vi "网络_构建url.vi"(10 "url":string, 11 "参数":string[](array[string])) -> (3 "结果url":string)   [LabVIEW 2014]
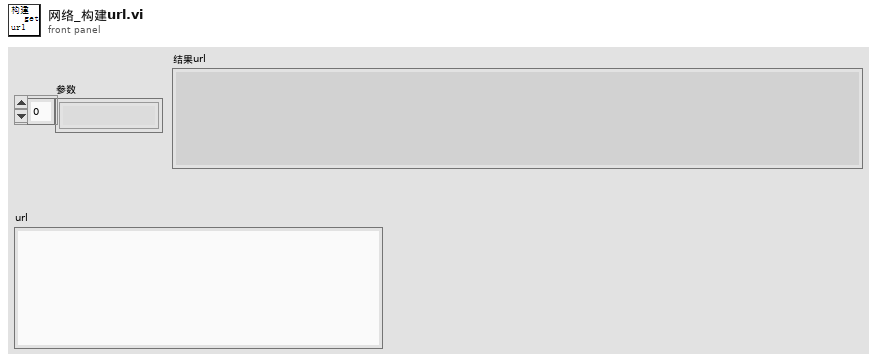
[diagram p1: front panel]
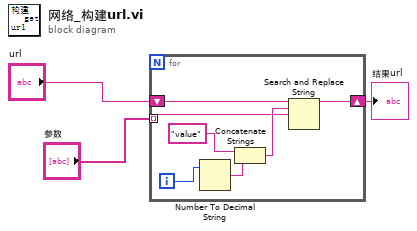
[diagram p0: block diagram]
diagram:
  n1 = for {
    tunnel: "参数" -> [w7] mode=indexing
    shift-right: [w6] -> w1
    shift-left: "url" -> [w5]
    i -> [w4]
    n2 = Number To Decimal String(number=w4) -> (decimal integer string=w9:string)  [unwired: 1 in]
    n3 = Concatenate Strings("value", w9) -> (w8:string)
    n4 = Search and Replace String(input string=w5, search string=w8, replace string=w7) -> (result string=w6:string)  [unwired: 5 in, 3 out]
  }
  "结果url" <- w1
